vi "ElectrodeAmplitude.vi"(8 "error in (no error)":errorcluster, 10 "Signal Amplitude":dbl=5.0 format="%#_2p", 11 "Electrode in":refnum<class "Electrode.lvclass">) -> (0 "error out":errorcluster, 3 "Electrode out":refnum<class "Electrode.lvclass">)   [LabVIEW 2012, in "Electrode.lvclass"]
uses:
  Electrode.lvclass
  Electrode.lvclass/Electrode.ctl
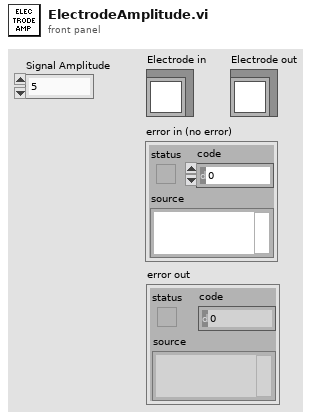
[diagram p1: front panel]
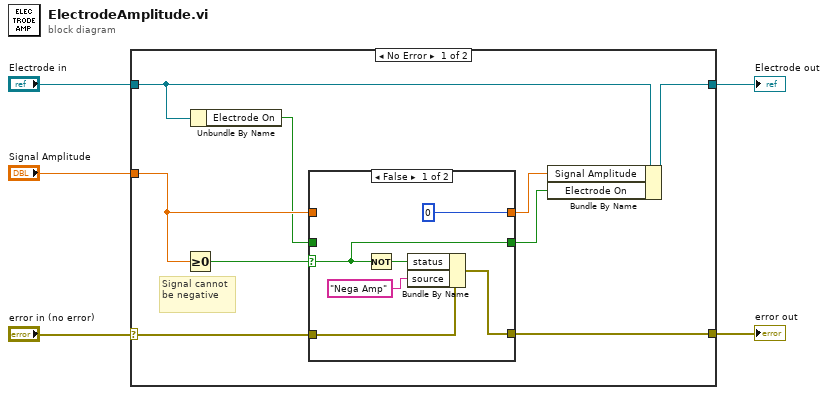
[diagram p0: block diagram]
diagram:
  n1 = case shown="No Error" "error in (no error)" {
    selector: "error in (no error)" -> [w7 w24]
    tunnel: [w6 w24] -> w4
    tunnel: [w14 w25] -> w2
    tunnel: "Electrode in" -> [w10 w25]
    tunnel: "Signal Amplitude" -> [w12 _]
    frame No Error {
      # "Signal cannot be negative"
      n2 = Greater Or Equal To 0?(x=w12) -> (x >= 0?=w13:bool)
      n3 = Unbundle By Name(w10) -> ("Electrode On"=w9:bool)
      n4 = case shown="False" w13 {
        selector: w13 -> [w16 _]
        tunnel: [w17 w21] -> w6
        tunnel: [0 w23] -> w11
        tunnel: w12 -> [_ w23]
        tunnel: w9 -> [_ w22]
        tunnel: [w16 w22] -> w8
        tunnel: w7 -> [w18 w21]
        frame False {
          n5 = Not(x=w16) -> (.not. x?=w19:bool)
          n6 = Bundle By Name(cluster=w18, "status"=w19, "source"="Nega Amp") -> (w17:errorcluster)
        }
        frame True {
        }
      }
      n7 = Bundle By Name(cluster=w10, "Signal Amplitude"=w11, "Electrode On"=w8) -> (w14:refnum<class "Electrode.lvclass">)
    }
    frame Error {
    }
  }
  "error out" <- w4
  "Electrode out" <- w2
